vi "GetMasterSerialIncoming2.vi"(7 "Master data ref":refnum<vi>, 8 "error in (no error)":errorcluster, 10 "Input buffer refnum":refnum<vi>, 11 "VISAResourceName in":refnum<vi>) -> (0 "error out":errorcluster)   [LabVIEW 2016]
panel:
  out "Data":u8[](array[numeric]) format="%x"
  # "Looks for incoming data on a serial port specified by the VISA refnum.\nIf an error would occur, a Stop-command is appended to the command \nqueue. To stop it, send TRUE to the Stop-notifier.\n\nSpecial version for incoming master-data\n\nMagne Lauritzen 2016"
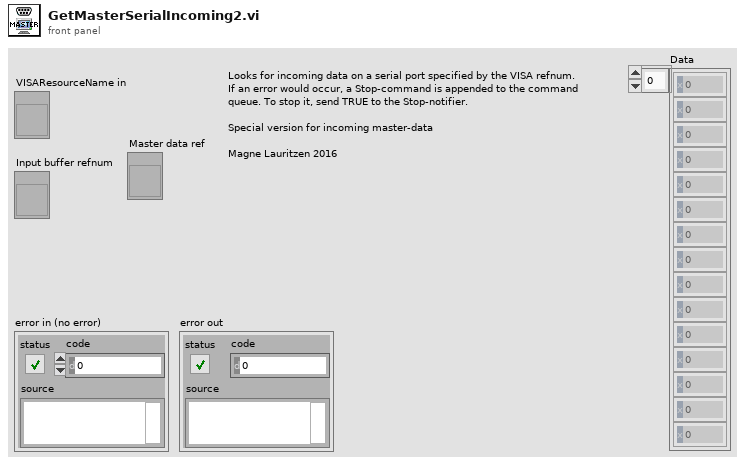
[diagram p1: front panel]
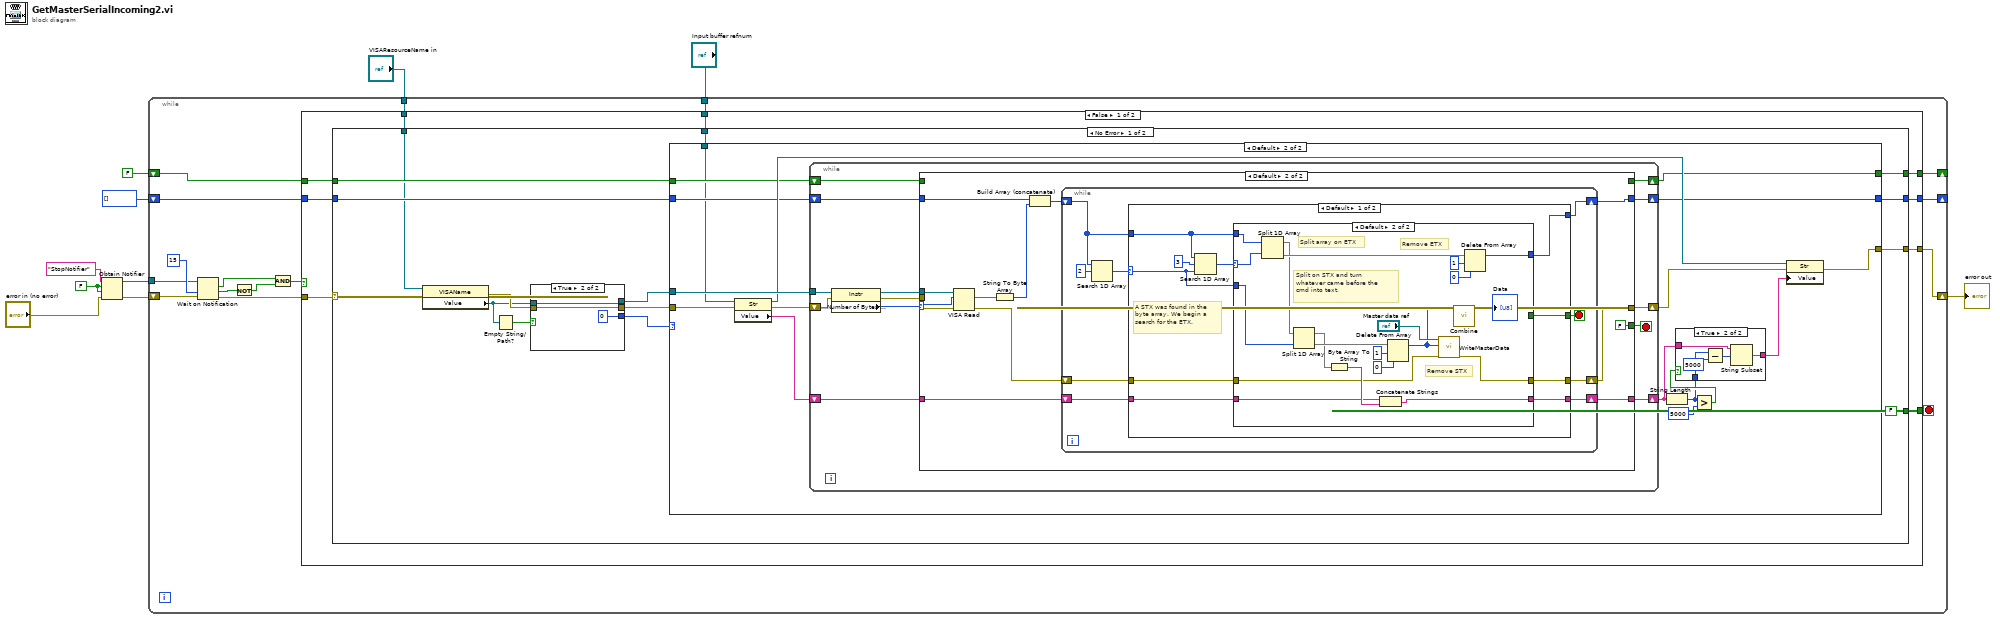
[diagram p0: block diagram]
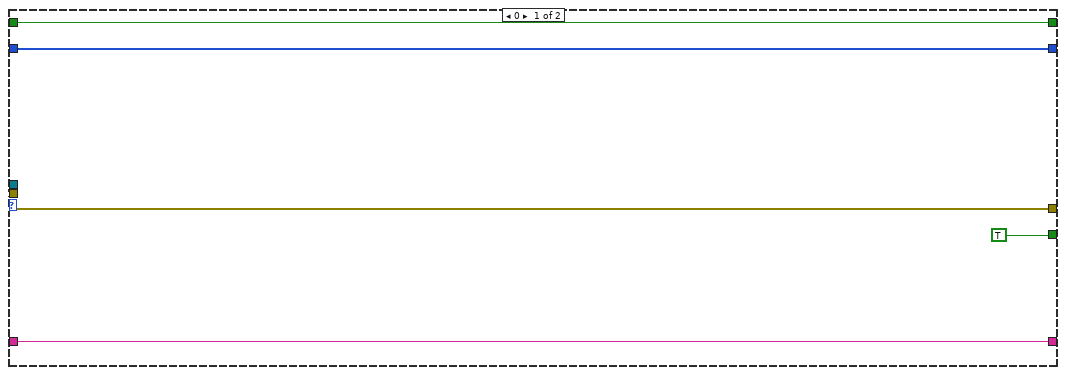
[diagram p4: hidden frame]
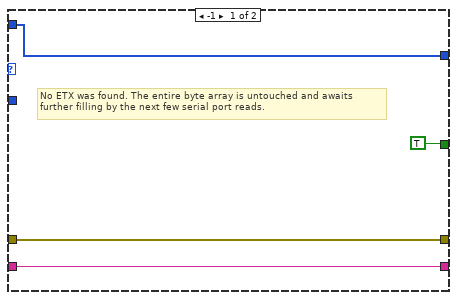
[diagram p5: hidden frame]
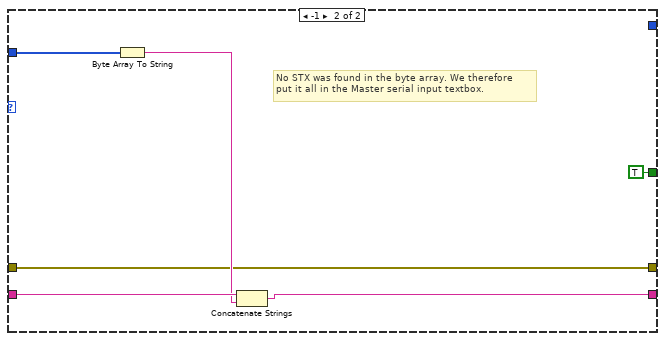
[diagram p6: hidden frame]
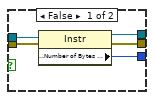
[diagram p7: hidden frame]
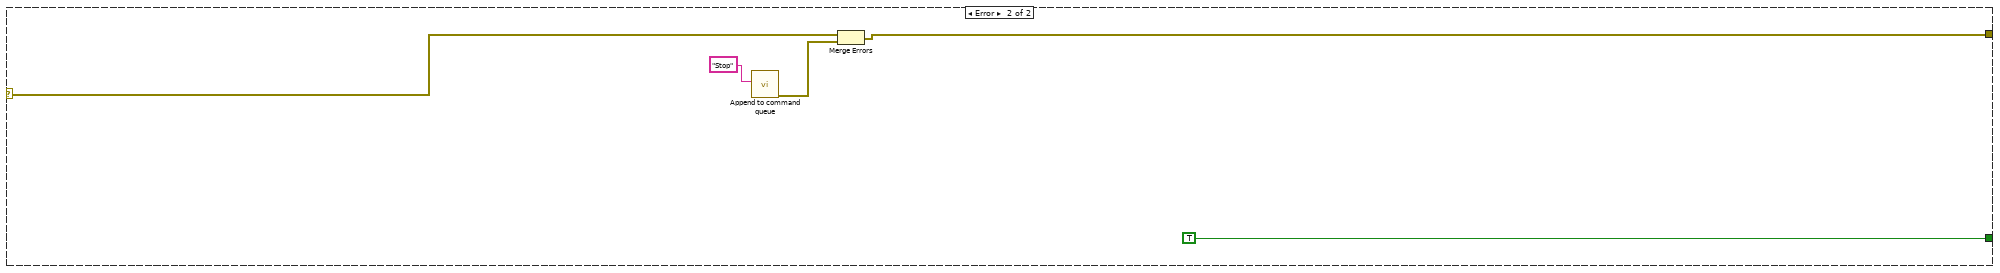
[diagram p8: hidden frame]
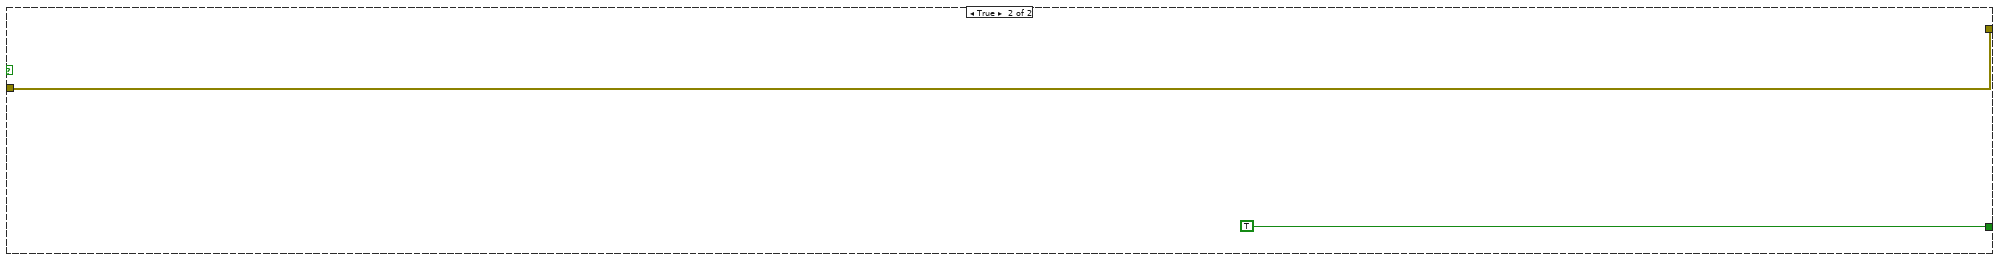
[diagram p9: hidden frame]
diagram:
  w7 = FALSE
  n1 = Obtain Notifier(name (unnamed)="StopNotifier", notification data type=w7, create if not found? (T)=w7, error in (no error)="error in (no error)") -> (notifier out=w5:refnum<notifier>, error out=w4:errorcluster)  [unwired: 1 out]
  n2 = while {
    shift-right: [w26] -> w10
    shift-left: w4 -> [w24]
    tunnel: w5 -> [w17]
    shift-right: [w15] -> _
    shift-left: FALSE -> [w16]
    shift-right: [w13] -> _
    shift-left: u8[] [] -> [w14]
    tunnel: "VISAResourceName in" -> [w12]
    tunnel: "Input buffer refnum" -> [w11]
    stop <- w18 stop-if-true
    n3 = Wait on Notification(notifier=w17, timeout in ms (-1)=u32 15 ("milliseconds to wait"), error in (no error)=w24) -> (notification=w21:bool, timed out?=w23:bool, error out=w19:errorcluster)  [unwired: 1 in, 1 out]
    n4 = Not(x=w23) -> (.not. x?=w22:bool)
    n5 = And(x=w21, y=w22) -> (x .and. y?=w20:bool)
    n6 = case shown="False" w20 {
      tunnel: [w35 w169] -> w26
      tunnel: w19 -> [w34 w169]
      tunnel: [w33 TRUE] -> w18
      tunnel: w16 -> [w32 _]
      tunnel: [w31 _] -> w15
      tunnel: w14 -> [w30 _]
      tunnel: [w29 _] -> w13
      tunnel: w12 -> [w28 _]
      tunnel: w11 -> [w27 _]
      frame False {
        n7 = case shown="No Error" w34 {
          selector: w34 -> [w45 w167]
          tunnel: [w46 w166] -> w35
          tunnel: [FALSE TRUE] -> w33
          tunnel: w32 -> [w41 _]
          tunnel: [w40 _] -> w31
          tunnel: w30 -> [w39 _]
          tunnel: [w38 _] -> w29
          tunnel: w28 -> [w37 _]
          tunnel: w27 -> [w36 _]
          frame No Error {
            n8 = property on="Property Node" class="VISAName"(reference=w37, error in=w45) -> (error out=w50:errorcluster, "Value"=w43:refnum<visa-resource-name>)  [unwired: 1 out]
            n9 = Empty String/Path?(string/path=w43) -> (empty?=w42:bool)
            n10 = case shown="True" w42 {
              tunnel: w50 -> [w160 w162]
              tunnel: [w159 u32 0 ("Bytes at Port")] -> w49
              tunnel: [w158 w161] -> w48
              tunnel: [w157 w162] -> w47
              tunnel: w43 -> [w156 w161]
              frame False {
                n11 = property class="Instr"(reference=w156, error in=w160) -> (reference out=w158:refnum<visa-resource-name>, error out=w157:errorcluster, "Serial Settings:Number of Bytes at Serial Port"=w159:u32)
              }
              frame True {
              }
            }
            n12 = case shown="Default" w49 {
              tunnel: w48 -> [_ w69]
              tunnel: w47 -> [w52 w64]
              tunnel: [w52 w67] -> w46
              tunnel: w41 -> [_ w62]
              tunnel: [_ w61] -> w40
              tunnel: w39 -> [w51 w60]
              tunnel: [w51 w59] -> w38
              tunnel: w36 -> [_ w58]
              frame 0 {
              }
              frame Default {
                n13 = property on="Property Node" class="Str"(reference=w58, error in=w64) -> (reference out=w63:refnum<vi>, error out=w65:errorcluster, "Value"=w66:string)
                n14 = while {
                  shift-right: [w85] -> w54
                  shift-left: w66 -> [w86]
                  shift-right: [w82] -> w68
                  shift-left: w65 -> [w81]
                  tunnel: w69 -> [w80]
                  shift-right: [w78] -> w61
                  shift-left: w62 -> [w79]
                  shift-right: [w76] -> w59
                  shift-left: w60 -> [w77]
                  stop <- w87 stop-if-true
                  n15 = property class="Instr"(reference=w80, error in=w81) -> (reference out=w84:refnum<visa-resource-name>, error out=w83:errorcluster, "Serial Settings:Number of Bytes at Serial Port"=w88:u32)
                  n16 = case shown="Default" w88 {
                    selector: w88 -> [_ w103]
                    tunnel: [TRUE FALSE] -> w87
                    tunnel: w86 -> [w92 w98]
                    tunnel: [w92 w97] -> w85
                    tunnel: w84 -> [_ w106]
                    tunnel: w83 -> [w91 w104]
                    tunnel: [w91 w94] -> w82
                    tunnel: w79 -> [w90 _]
                    tunnel: [w90 _] -> w78
                    tunnel: w77 -> [w89 w101]
                    tunnel: [w89 w96] -> w76
                    frame 0 {
                    }
                    frame Default {
                      n17 = VISA Read(VISA resource name=w106, byte count=w103, error in (no error)=w104) -> (read buffer=w102:string, error out=w95:errorcluster)  [unwired: 2 out]
                      n18 = String To Byte Array(string=w102) -> (unsigned byte array=w100:u8[])
                      n19 = Build Array (concatenate)(w101, w100) -> (w99:u8[])
                      n20 = while {
                        shift-right: [w110] -> w96
                        shift-left: w99 -> [w114]
                        shift-right: [w112] -> w97
                        shift-left: w98 -> [w113]
                        shift-right: [w108] -> w94
                        shift-left: w95 -> [w109]
                        stop <- w107 stop-if-true
                        n21 = Search 1D Array(1D array=w114, element=u8 2) -> (index of element=w111:i32)  [unwired: 1 in]
                        n22 = case shown="Default" w111 {
                          selector: w111 -> [w122 _]
                          tunnel: w114 -> [w123 w155]
                          tunnel: w113 -> [w120 w154]
                          tunnel: [w119 w152] -> w112
                          tunnel: [w121 _] -> w110
                          tunnel: [w118 w151] -> w108
                          tunnel: w109 -> [w117 w151]
                          tunnel: [w116 TRUE] -> w107
                          frame Default {
                            # "A STX was found in the \nbyte array. We begin a \nsearch for the ETX."
                            n23 = Search 1D Array(1D array=w123, element=u8 3, start index (0)=w122) -> (index of element=w124:i32)
                            n24 = case shown="Default" w124 {
                              selector: w124 -> [_ w148]
                              tunnel: w123 -> [w129 w149]
                              tunnel: w122 -> [_ w142]
                              tunnel: [w129 w144] -> w121
                              tunnel: w120 -> [w128 w136]
                              tunnel: [w128 w135] -> w119
                              tunnel: [w127 w131] -> w118
                              tunnel: w117 -> [w127 w130]
                              tunnel: [TRUE _] -> w116
                              frame -1 {
                                # "No ETX was found. The entire byte array is untouched and awaits \nfurther filling by the next few serial port reads."
                              }
                              frame Default {
                                # "Remove STX"
                                # "Split on STX and turn whatever came before the cmd into text."
                                # "Split array on ETX"
                                # "Remove ETX"
                                n25 = Split 1D Array(array=w149, index=w148) -> (first subarray=w143:u8[], second subarray=w147:u8[])
                                n26 = Split 1D Array(array=w143, index=w142) -> (first subarray=w138:u8[], second subarray=w139:u8[])
                                n27 = Byte Array To String(unsigned byte array=w138) -> (string=w137:string)
                                n28 = Concatenate Strings(w136, w137) -> (w135:string)
                                n29 = Delete From Array(array=w139, length=1, index=0) -> (array with subset deleted=w132:u8[])  [unwired: 1 out]
                                n30 = call "WriteMasterData.vi"("error in (no error)"=w130, "New data"=w132, "Array in"="Master data ref") -> ("error out"=w131:errorcluster)  [unwired: 8 in]
                                n31 = call "Combine.vi"("NewVal"=w132) -> ("Data"=→"Data":u8[])  [unwired: 10 in]
                                n32 = Delete From Array(array=w147, length=1, index=0) -> (array with subset deleted=w144:u8[])  [unwired: 1 out]
                              }
                            }
                          }
                          frame -1 {
                            # "No STX was found in the byte array. We therefore\nput it all in the Master serial input textbox."
                            n33 = Byte Array To String(unsigned byte array=w155) -> (string=w153:string)
                            n34 = Concatenate Strings(w154, w153) -> (w152:string)
                          }
                        }
                      }
                    }
                  }
                }
                n35 = String Length(string=w54) -> (length=w55:i32)
                n36 = Greater?(x=w55, y=5000) -> (0:w56:bool)
                n37 = case shown="True" w56 {
                  tunnel: w55 -> [_ w75]
                  tunnel: w54 -> [w70 w72]
                  tunnel: [w70 w71] -> w53
                  frame False {
                  }
                  frame True {
                    n38 = Subtract(x=w75, y=5000) -> (x-y=w73:i32)
                    n39 = String Subset(string=w72, offset (0)=w73) -> (substring=w71:string)  [unwired: 1 in]
                  }
                }
                n40 = property on="Property Node" class="Str"(reference=w63, error in=w68, "Value"=w53) -> (error out=w67:errorcluster)  [unwired: 1 out]
              }
            }
          }
          frame Error {
            n41 = call "Append to command queue.vi"("Single command"="Stop") -> ("error out"=w165:errorcluster)  [unwired: 10 in]
            n42 = Merge Errors(w167, w165) -> (w166:errorcluster)
          }
        }
      }
      frame True {
      }
    }
  }
  "error out" <- w10
